vi "calibratePlatforms.vi"() -> ()   [LabVIEW 2017]
doc: "The load cells output a voltage even when no weight is present on the platform. This needs to be measured so that it can be subtracted from subsequent measurements of platform load. The VI will output a spreadsheet saved in the current folder."
uses:
  <vilib>/Utility/file.llb/Write Delimited Spreadsheet (DBL).vi
  <vilib>/Utility/file.llb/Write Delimited Spreadsheet (string).vi
panel:
  in  "mazeDirection":string(combo)="clockwise"
  out "load cell\nsignal":dbl[](array[numeric])
  out "index":i32[](array[numeric])
  out "badChannels":string[](array[string])
  out "bad platforms":i32[](array[numeric])
  out "names out":string[](array[string])
  out "x/y":dbl[](array[numeric])
  in  "stop 2":bool
  in  "50 g":bool
  in  "Zero":bool
  # "1. First zero the platforms\n2. Place 50 g weights on platforms\n3. Run 50 g calibration"
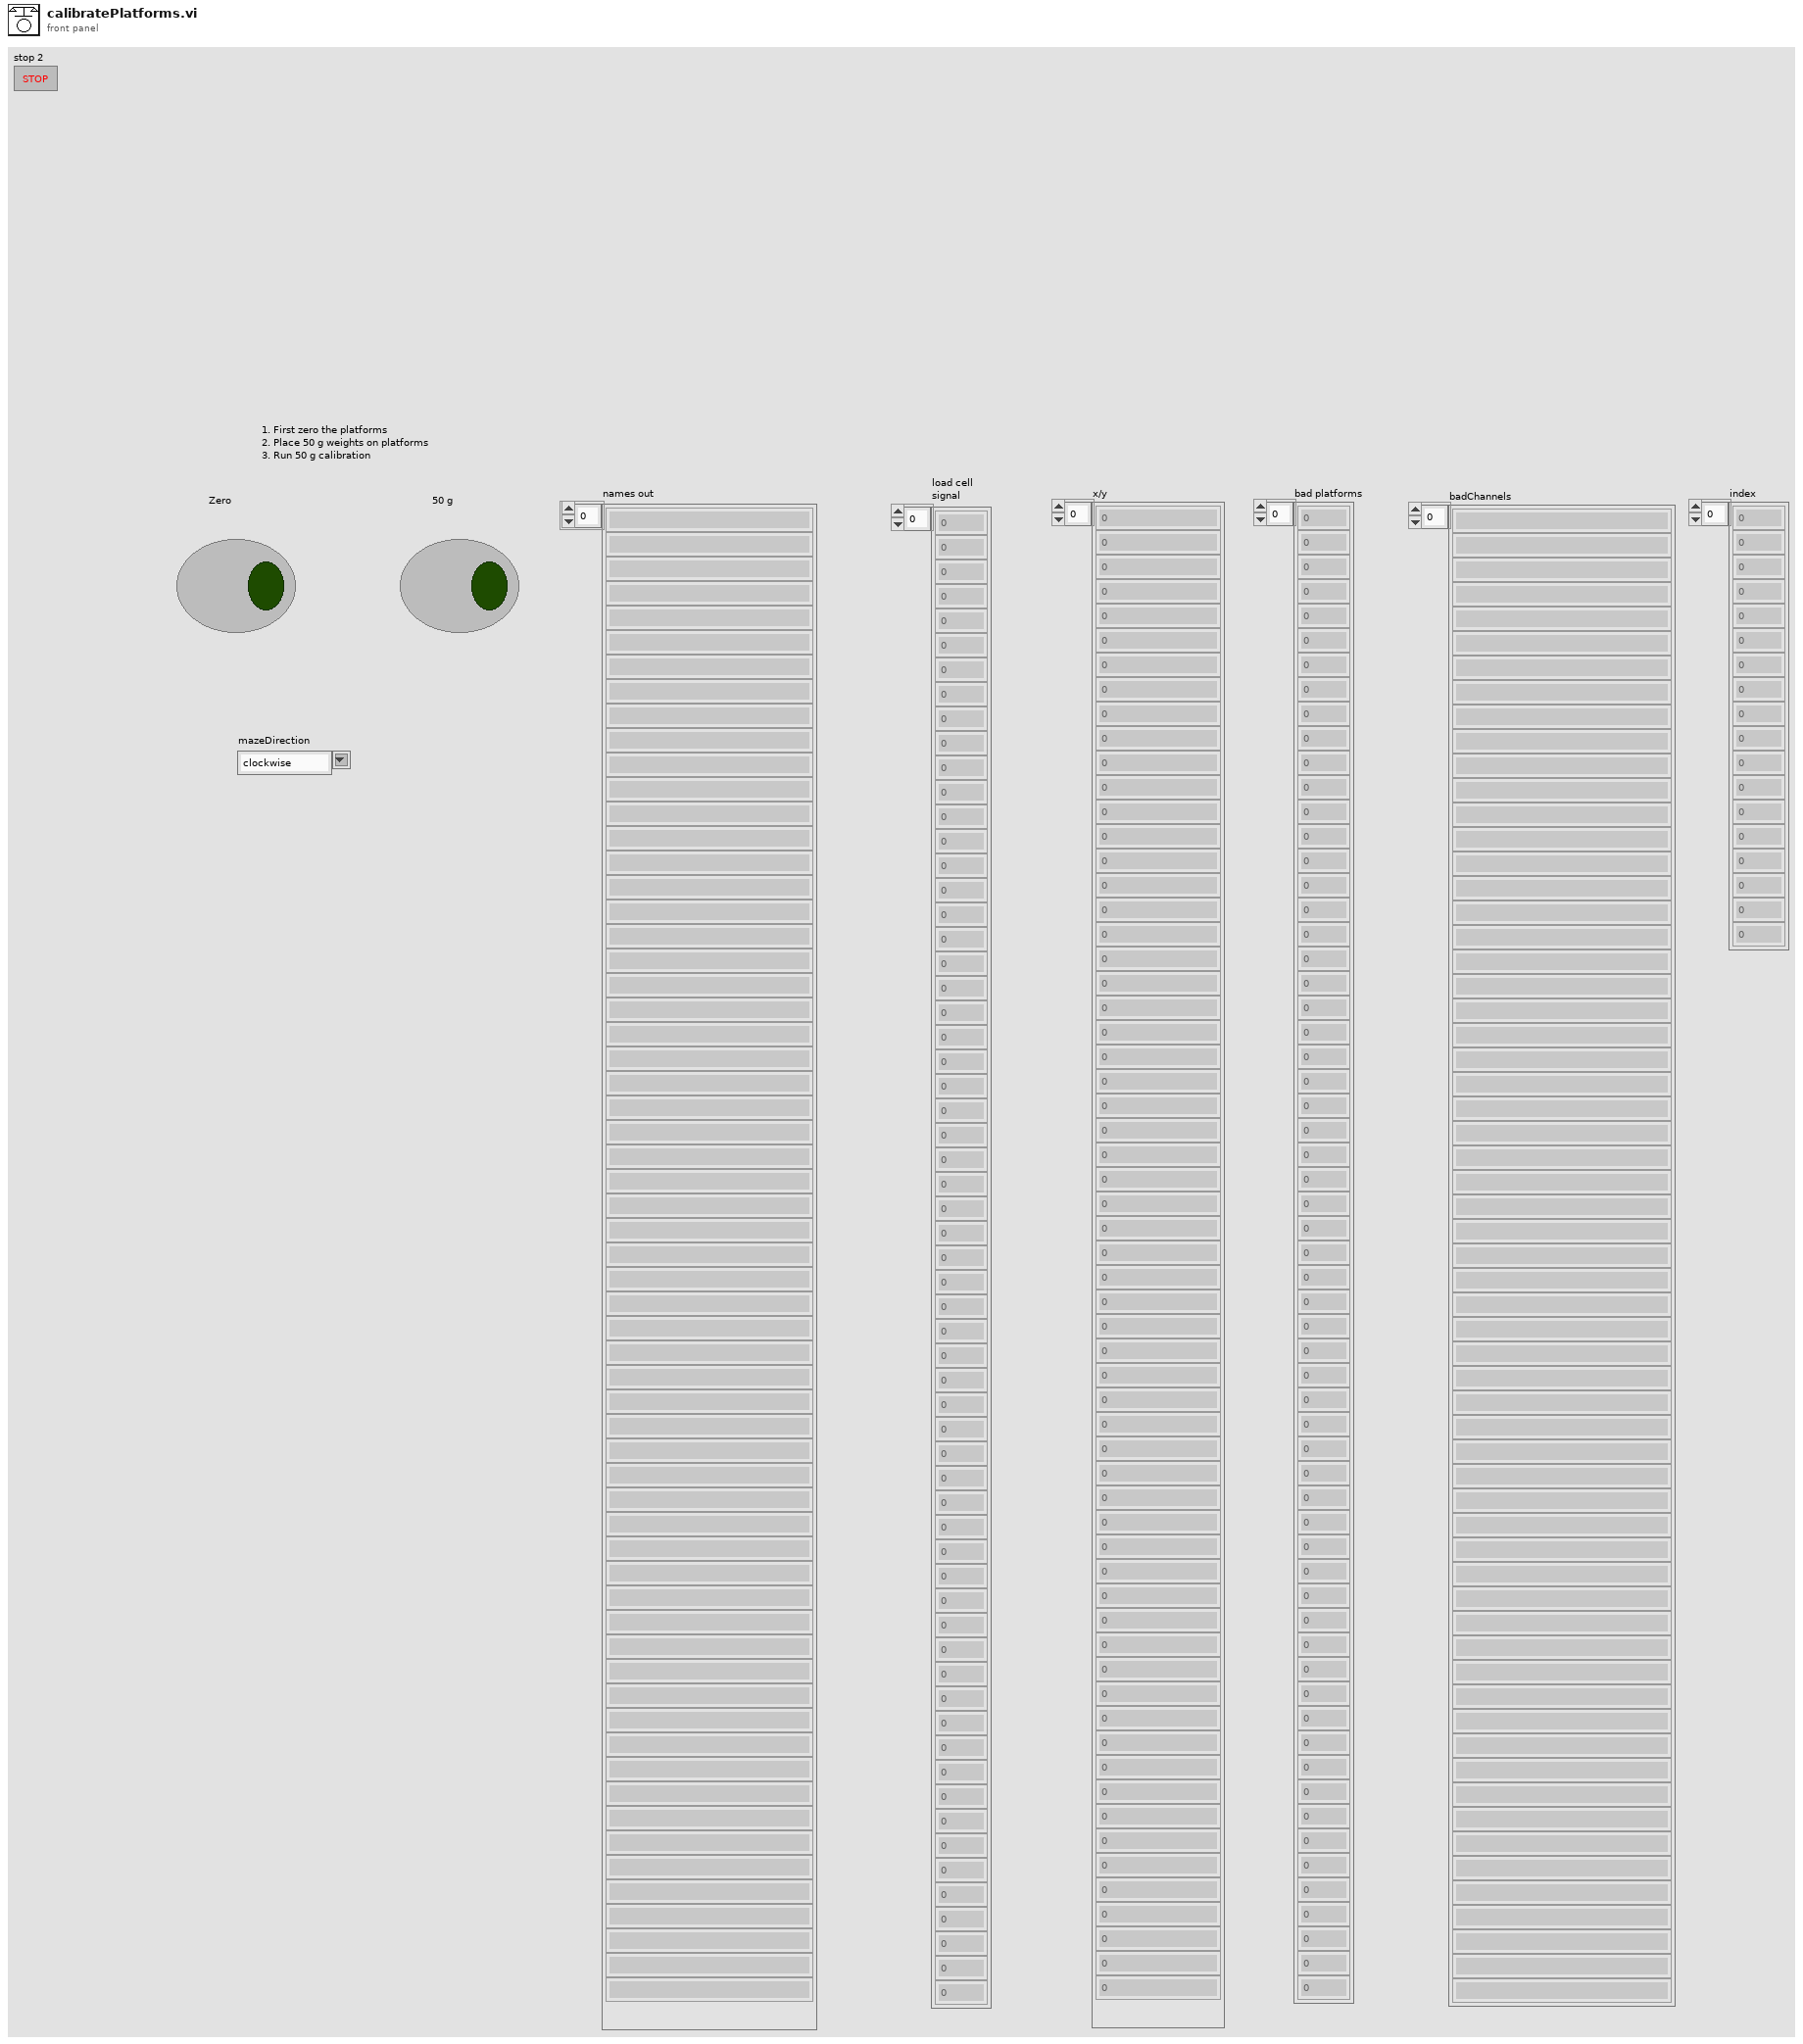
[diagram p1: front panel]
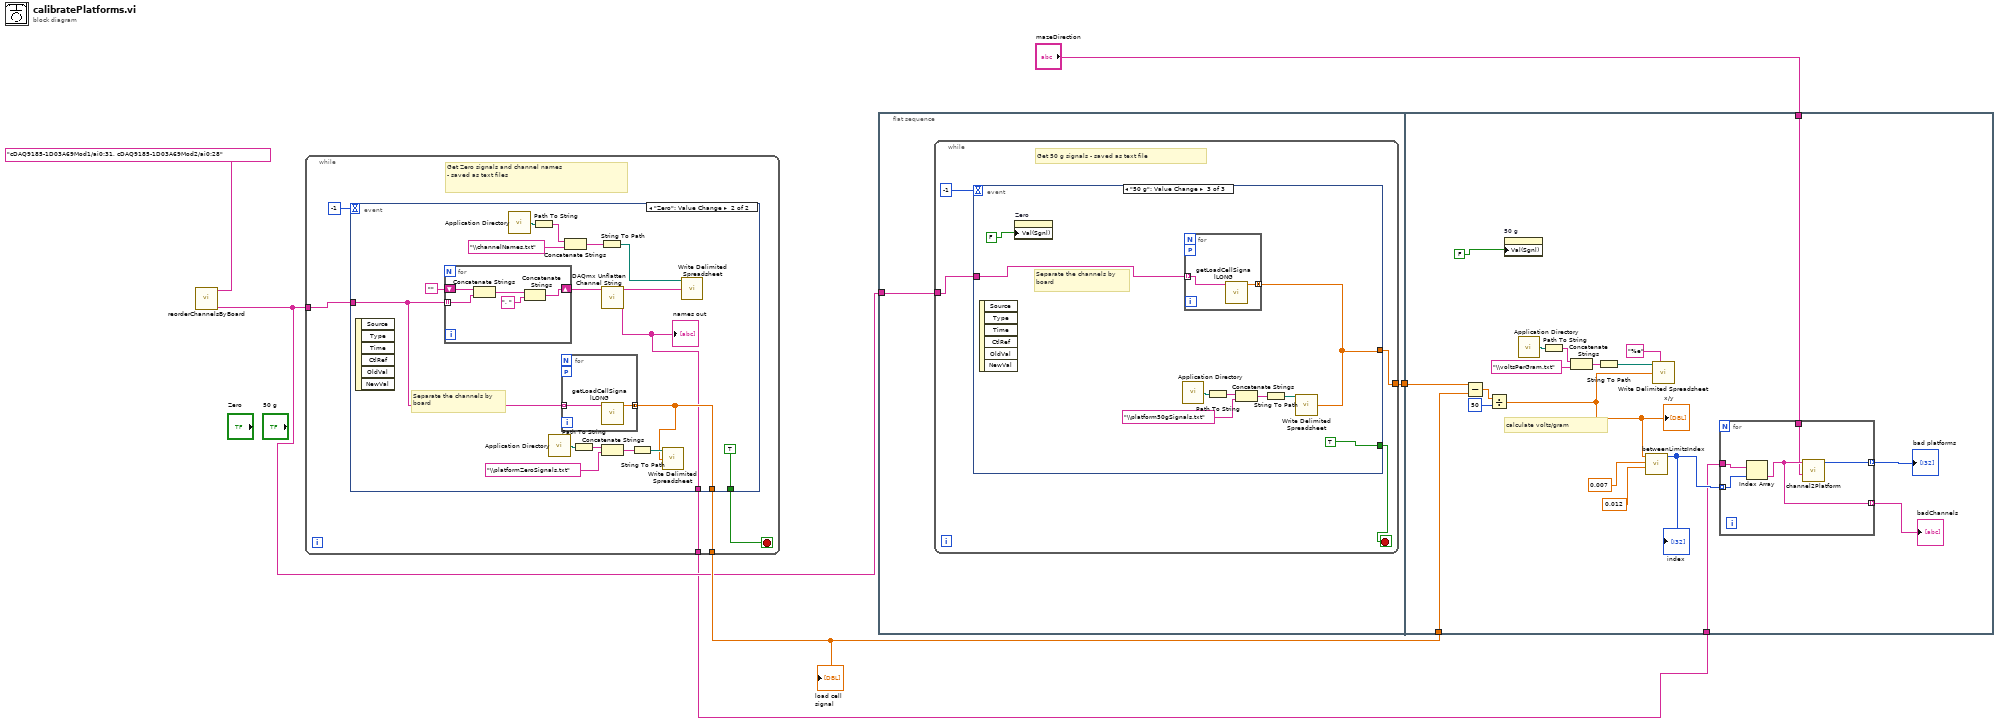
[diagram p0: block diagram]
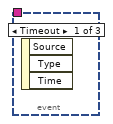
[diagram p2: hidden frame]
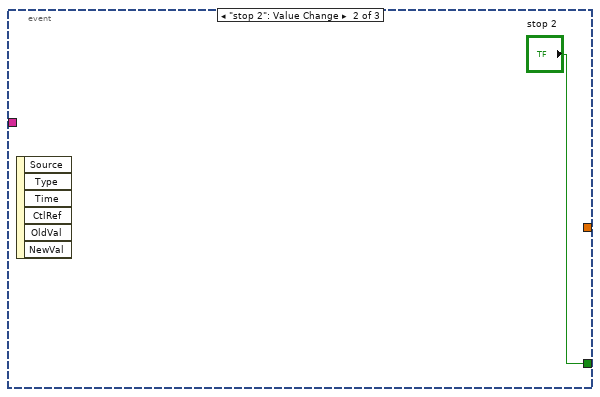
[diagram p3: hidden frame]
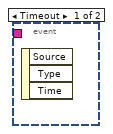
[diagram p4: hidden frame]
diagram:
  n1 = call "reorderChannelsByBoard.vi"("DAQmx \nPhysical Channel"=tag "cDAQ9185-1D03A69Mod1/ai0:31, cDAQ9185-1D03A69Mod2/ai0:28" ("DAQmx \nPhysical Channel")) -> ("Separated inputs\nas strings"=w3:string[])  [unwired: 8 in, 2 out]
  n2 = while {
    tunnel: w3 -> [w10]
    tunnel: [w8] -> w4
    tunnel: [w7] -> w2
    stop <- w9 stop-if-true
    # "Get Zero signals and channel names \n- saved as text files"
    n3 = event shown="[1] \"Zero\": Value Change" {
      selector: _ -> [_ _]
      dyn-events: _ -> [_ _]
      timeout: -1 -> [_ _]
      tunnel: w10 -> [_ w15]
      tunnel: [_ w14] -> w8
      tunnel: [_ TRUE] -> w9
      tunnel: [_ w12] -> w7
      event Timeout {
        n4 = event-data() -> ()  [unwired: 1 in, 3 out]
      }
      event "Zero": Value Change {
        # "Separate the channels by\nboard"
        n5 = event-data() -> ()  [unwired: 1 in, 6 out]
        n6 = for {
          shift-right: [w31] -> w26
          shift-left: "" -> [w32]
          tunnel: w15 -> [w28] mode=indexing
          n7 = Concatenate Strings(w32, w28) -> (w30:string)
          n8 = Concatenate Strings(w30, ", ") -> (w31:string)
        }
        n9 = call <vilib>:"Application Directory.vi"() -> ("Application Directory"=w24:path)
        n10 = Path To String(path=w24) -> (string=w23:string)
        n11 = call <vilib>:"Application Directory.vi"() -> ("Application Directory"=w19:path)
        n12 = for {
          workers-P: _ -> [_]
          tunnel: [w33] -> w14 mode=concatenating
          tunnel: w15 -> [w34] mode=indexing
          n13 = call "getLoadCellSignalLONG.vi"("DAQmx Physical Channel"=w34) -> ("load cell\nsignal"=w33:dbl[])  [unwired: 10 in]
        }
        n14 = Concatenate Strings(w23, "\\channelNames.txt") -> (w22:string)
        n15 = Path To String(path=w19) -> (string=w18:string)
        n16 = String To Path(string=w22) -> (path=w21:path)
        n17 = call <vilib>:"DAQmx Unflatten Channel String.vi"("names in"=w26) -> ("names out"=w12:string[])  [unwired: 13 in, 1 out]
        "names out" <- w12
        n18 = Concatenate Strings(w18, "\\platformZeroSignals.txt") -> (w17:string)
        n19 = String To Path(string=w17) -> (path=w16:path)
        n20 = call-poly <vilib>:"Write Delimited Spreadsheet.vi"("file path (dialog if empty)"=w16, "1D data"=w14) -> ()  [unwired: 12 in, 2 out]
        n21 = call-poly <vilib>:"Write Delimited Spreadsheet.vi"("file path (dialog if empty)"=w21, "1D data"=w12) -> ()  [unwired: 12 in, 2 out]
      }
    }
  }
  "load cell\nsignal" <- w4
  n22 = flat-sequence {
    tunnel: w3 -> [w35]
    tunnel: [w36] -> w5
    tunnel: w5 -> [w62]
    tunnel: w4 -> [w63]
    tunnel: w2 -> [w56]
    tunnel: "mazeDirection" -> [w53]
    frame #0 {
      n23 = while {
        tunnel: [w39] -> w36
        tunnel: w35 -> [w37]
        stop <- w38 stop-if-true
        # "Get 50 g signals - saved as text file"
        n24 = event shown="[2] \"50 g\": Value Change" {
          selector: _ -> [_ _ _]
          dyn-events: _ -> [_ _ _]
          timeout: -1 -> [_ _ _]
          tunnel: [_ "stop 2" TRUE] -> w38
          tunnel: [_ _ w44] -> w39
          tunnel: w37 -> [_ _ w42]
          event Timeout {
            n25 = event-data() -> ()  [unwired: 1 in, 3 out]
          }
          event "stop 2": Value Change {
            n26 = event-data() -> ()  [unwired: 1 in, 6 out]
          }
          event "50 g": Value Change {
            # "Separate the channels by\nboard"
            n27 = event-data() -> ()  [unwired: 1 in, 6 out]
            n28 = property on="Zero" class="Bool (strict)"("Val(Sgnl)"=FALSE) -> ()  [unwired: 2 in, 2 out]
            n29 = call <vilib>:"Application Directory.vi"() -> ("Application Directory"=w49:path)
            n30 = for {
              workers-P: _ -> [_]
              tunnel: [w52] -> w44 mode=concatenating
              tunnel: w42 -> [w51] mode=indexing
              n31 = call "getLoadCellSignalLONG.vi"("DAQmx Physical Channel"=w51) -> ("load cell\nsignal"=w52:dbl[])  [unwired: 10 in]
            }
            n32 = Path To String(path=w49) -> (string=w48:string)
            n33 = Concatenate Strings(w48, "\\platform50gSignals.txt") -> (w47:string)
            n34 = String To Path(string=w47) -> (path=w46:path)
            n35 = call-poly <vilib>:"Write Delimited Spreadsheet.vi"("file path (dialog if empty)"=w46, "1D data"=w44) -> ()  [unwired: 12 in, 2 out]
          }
        }
      }
    }
    frame #1 {
      # "calculate volts/gram"
      n36 = Subtract(x=w62, y=w63) -> (x-y=w67:dbl[])
      n37 = Divide(x=w67, y=50) -> (x/y=w60:dbl[])
      "x/y" <- w60
      n38 = property on="50 g" class="Bool (strict)"("Val(Sgnl)"=FALSE) -> ()  [unwired: 2 in, 2 out]
      n39 = call <vilib>:"Application Directory.vi"() -> ("Application Directory"=w68:path)
      n40 = Path To String(path=w68) -> (string=w69:string)
      n41 = Concatenate Strings(w69, "\\voltsPerGram.txt") -> (w70:string)
      n42 = String To Path(string=w70) -> (path=w71:path)
      n43 = call "betweenLimitsIndex.vi"("upper limit"=0.012, "lower limit"=0.007, "Data"=w60) -> ("index"=w57:i32[])  [unwired: 8 in]
      "index" <- w57
      n44 = call-poly <vilib>:"Write Delimited Spreadsheet.vi"("file path (dialog if empty)"=w71, "format (%.3f)"="%e", "1D data"=w60) -> ()  [unwired: 11 in, 2 out]
      n45 = for {
        tunnel: w57 -> [w76] mode=indexing
        tunnel: w56 -> [w75]
        tunnel: [w74] -> w55 mode=indexing
        tunnel: [w73] -> w54 mode=indexing
        tunnel: w53 -> [w72]
        n46 = Index Array(array=w75, index=w76) -> (element=w73:string)
        n47 = call "channel2Platform.vi"("mazeDirection"=w72, "DAQmx \nPhysical Channel"=w73) -> ("Platform number"=w74:i32)  [unwired: 9 in]
      }
      "bad platforms" <- w55
      "badChannels" <- w54
    }
  }
